vi "USBL_Test.vi"() -> ()   [LabVIEW 2017]
uses:
  <vilib>/Utility/error.llb/DialogType.ctl
  <vilib>/DAQmx/write.llb/DAQmx Write (Analog Wfm 1Chan NSamp).vi
  <vilib>/DAQmx/read.llb/DAQmx Read (Analog 1D Wfm NChan NSamp).vi
  <vilib>/DAQmx/create/channels.llb/DAQmx Create Channel (AO-Voltage-Basic).vi
  <vilib>/DAQmx/configure/events/hardwareSignals.llb/DAQmx Export Signal (Most Signals).vi
  <vilib>/DAQmx/configure/timing.llb/DAQmx Timing (Sample Clock).vi
  <vilib>/DAQmx/miscellaneous.llb/DAQmx Fill In Error Info.vi
  <vilib>/DAQmx/create/channels.llb/DAQmx Create Channel (AI-Voltage-Basic).vi
  <vilib>/DAQmx/configure/trigger.llb/DAQmx Start Trigger (Digital Edge).vi
  <vilib>/Analysis/NI_AALBase.lvlib
panel:
  out "Rx. Signal 9":waveform(dbl)(graph)={"t0"=timestamp(0 s since 1904-01-01), "dt"=1e-05, "Y"=array[100000 elements]}
  out "Rx. Signal 8":waveform(dbl)(graph)={"t0"=timestamp(0 s since 1904-01-01), "dt"=1e-05, "Y"=array[100000 elements]}
  out "Rx. Signal 7":waveform(dbl)(graph)={"t0"=timestamp(0 s since 1904-01-01), "dt"=1e-05, "Y"=array[100000 elements]}
  out "Rx. Signal 6":waveform(dbl)(graph)={"t0"=timestamp(0 s since 1904-01-01), "dt"=1e-05, "Y"=array[100000 elements]}
  out "Rx. Signal 5":waveform(dbl)(graph)={"t0"=timestamp(0 s since 1904-01-01), "dt"=1e-05, "Y"=array[100000 elements]}
  out "Rx. Signal 4":waveform(dbl)(graph)={"t0"=timestamp(0 s since 1904-01-01), "dt"=1e-05, "Y"=array[100000 elements]}
  out "Rx. Signal 3":waveform(dbl)(graph)={"t0"=timestamp(0 s since 1904-01-01), "dt"=1e-05, "Y"=array[100000 elements]}
  out "Rx. Signal 2":waveform(dbl)(graph)={"t0"=timestamp(0 s since 1904-01-01), "dt"=1e-05, "Y"=array[100000 elements]}
  in  "Tx.Channel":tag="PXI1Slot12/ao1"
  in  "Trigger Output":tag="/PXI1Slot12/PFI2"
  in  "Frequency (Hz)":dbl=5000.0
  in  "Amplitude  (V)":dbl=2.5
  in  "Pulse Length (sec)":dbl=0.1
  in  "Device 2":tag="PXI1Slot12"
  out "Rx. Signal":waveform(dbl)[](graph)=[{"t0"=timestamp(3673929480.9649253 s since 1904-01-01), "dt"=9.999999999999972e-06, "Y"=array[10000 elements], "attributes"=variant("NI_ChannelName"=variant(string "PXI1Slot16/ai0"), "NI_UnitDescription"=variant(string "Volts"))}, {"t0"=timestamp(3673929480.9649253 s since 1904-01-01), "dt"=9.999999999999972e-06, "Y"=array[10000 elements], "attributes"=variant("NI_ChannelName"=variant(string "PXI1Slot16/ai1"), "NI_UnitDescription"=variant(string "Volts"))}, {"t0"=timestamp(3673929480.9649253 s since 1904-01-01), "dt"=9.999999999999972e-06, "Y"=array[10000 elements], "attributes"=variant("NI_ChannelName"=variant(string "PXI1Slot16/ai2"), "NI_UnitDescription"=variant(string "Volts"))}, {"t0"=timestamp(3673929480.9649253 s since 1904-01-01), "dt"=9.999999999999972e-06, "Y"=array[10000 elements], "attributes"=variant("NI_ChannelName"=variant(string "PXI1Slot16/ai3"), "NI_UnitDescription"=variant(string "Volts"))}, {"t0"=timestamp(3673929480.9649253 s since 1904-01-01), "dt"=9.999999999999972e-06, "Y"=array[10000 elements], "attributes"=variant("NI_ChannelName"=variant(string "PXI1Slot16/ai4"), "NI_UnitDescription"=variant(string "Volts"))}, {"t0"=timestamp(3673929480.9649253 s since 1904-01-01), "dt"=9.999999999999972e-06, "Y"=array[10000 elements], "attributes"=variant("NI_ChannelName"=variant(string "PXI1Slot16/ai5"), "NI_UnitDescription"=variant(string "Volts"))}, {"t0"=timestamp(3673929480.9649253 s since 1904-01-01), "dt"=9.999999999999972e-06, "Y"=array[10000 elements], "attributes"=variant("NI_ChannelName"=variant(string "PXI1Slot16/ai6"), "NI_UnitDescription"=variant(string "Volts"))}, {"t0"=timestamp(3673929480.9649253 s since 1904-01-01), "dt"=9.999999999999972e-06, "Y"=array[10000 elements], "attributes"=variant("NI_ChannelName"=variant(string "PXI1Slot16/ai7"), "NI_UnitDescription"=variant(string "Volts"))}]
  in  "Number of Sample":i32=10000
  in  "Rx.Time Length (sec)":dbl=1.0
  in  "Trigger Input":tag="/PXI1Slot12/PFI2"
  in  "Sampling Frequency (Hz)":dbl=100000.0
  in  "Rx.Channel":tag="PXI1Slot16/ai0:7"
  in  "Device":tag="PXI1Slot16"
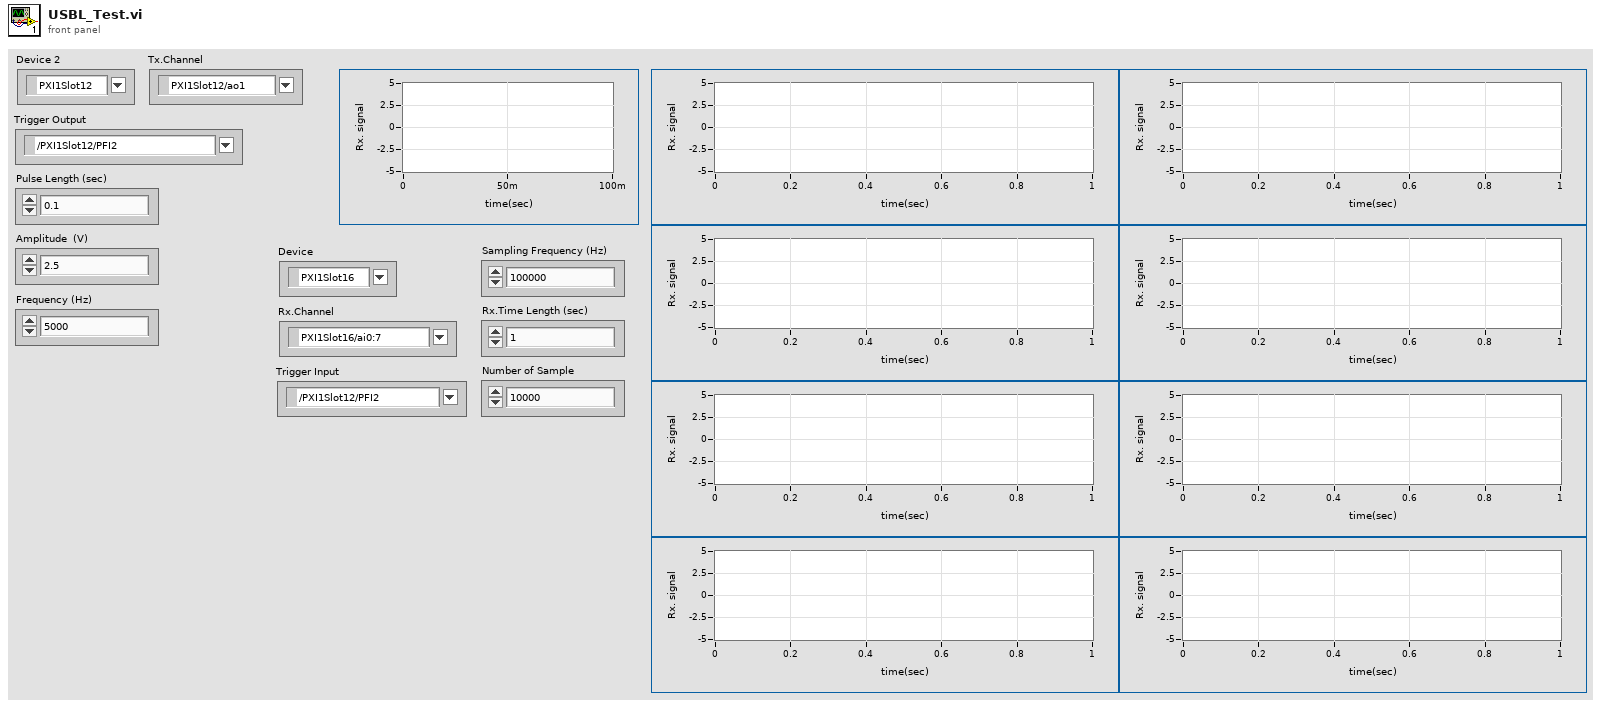
[diagram p1: front panel]
types:
  T1 = typedef "DialogType.ctl" = u16
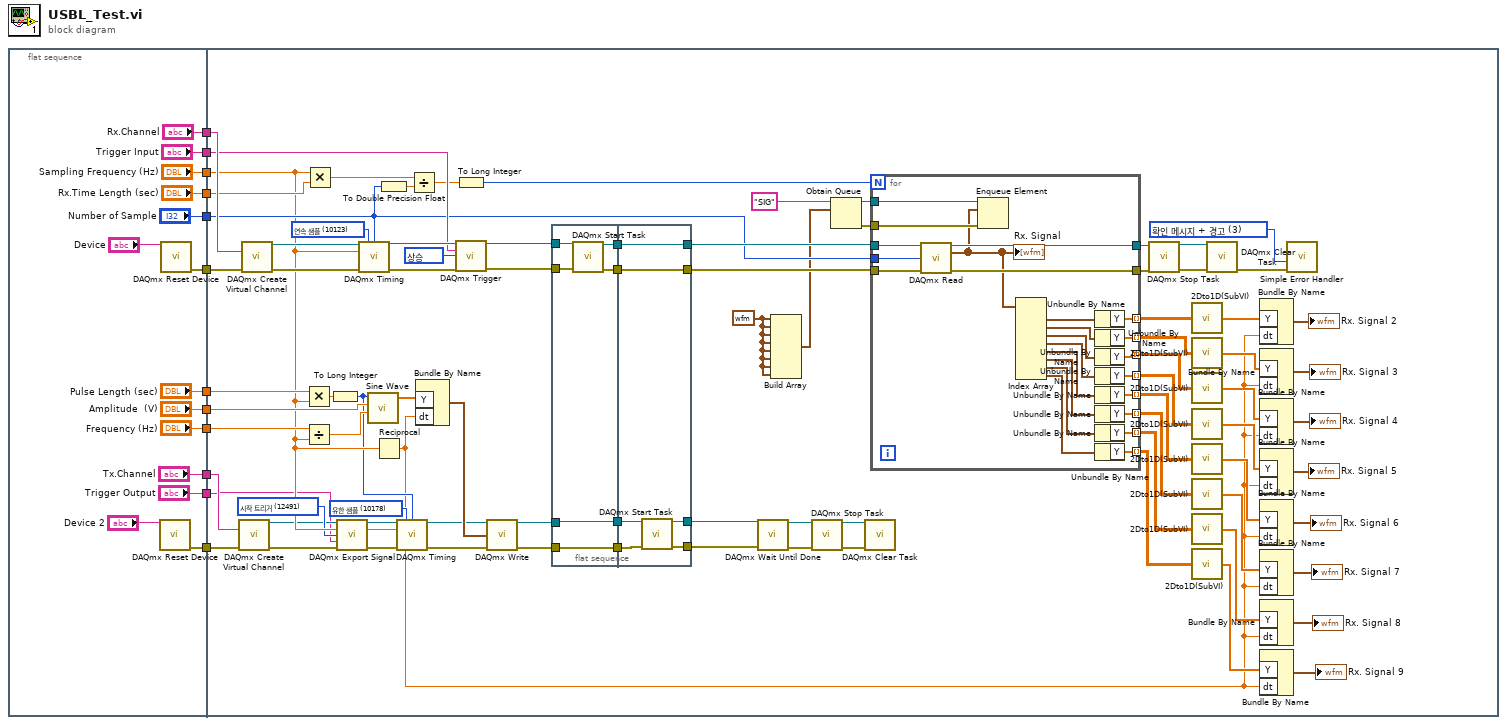
[diagram p0: block diagram]
diagram:
  n1 = flat-sequence {
    tunnel: [w25] -> w12
    tunnel: ["Rx.Channel"] -> w11
    tunnel: ["Trigger Input"] -> w10
    tunnel: ["Sampling Frequency (Hz)"] -> w9
    tunnel: ["Rx.Time Length (sec)"] -> w8
    tunnel: ["Number of Sample"] -> w7
    tunnel: [w18] -> w6
    tunnel: ["Pulse Length (sec)"] -> w5
    tunnel: ["Amplitude  (V)"] -> w4
    tunnel: ["Frequency (Hz)"] -> w3
    tunnel: ["Tx.Channel"] -> w2
    tunnel: ["Trigger Output"] -> w1
    tunnel: w12 -> [w84]
    tunnel: w11 -> [w111]
    tunnel: w10 -> [w108]
    tunnel: w9 -> [w75]
    tunnel: w8 -> [w110]
    tunnel: w7 -> [w97]
    tunnel: w6 -> [w83]
    tunnel: w5 -> [w80]
    tunnel: w4 -> [w79]
    tunnel: w3 -> [w78]
    tunnel: w2 -> [w73]
    tunnel: w1 -> [w63]
    frame #0 {
      n2 = call <vilib>:"DAQmx Reset Device.vi"("device in"="Device 2") -> ("error out"=w18:errorcluster)  [unwired: 14 in]
      n3 = call <vilib>:"DAQmx Reset Device.vi"("device in"="Device") -> ("error out"=w25:errorcluster)  [unwired: 14 in]
    }
    frame #1 {
      w72 = 12491 items=["AI 변환 클럭"=12484, "10MHz 참조 클럭"=12536, "20MHz 타임베이스 클럭"=12486, "샘플 클럭"=12487, "진행 트리거"=12488, "참조 트리거"=12490, "시작 트리거"=12491, "진행 완료 이벤트"=12492, "AI 홀드 완료 이벤트"=12493, "카운터 출력 이벤트"=12494, "변경 감지 이벤트"=12511, "워치독 타이머 만료 이벤트"=12512] ("signal")
      w82 = 10178 items=["유한 샘플"=10178, "연속 샘플"=10123, "하드웨어 타이밍에 의한 단일 포인트"=12522] ("sample mode")
      w87 = T1 3 items=["대화 상자 없음", "확인 메시지", "메시지 지속 또는 정지", "확인 메시지 + 경고", "지속/정지 + 경고"] ("대화 상자 타입 (확인 메시지:1)")
      w92 = waveform(dbl) {"t0"=timestamp(0 s since 1904-01-01), "dt"=1.0, "Y"=[]} ("Waveform")
      w101 = 10123 items=["유한 샘플"=10178, "연속 샘플"=10123, "하드웨어 타이밍에 의한 단일 포인트"=12522] ("sample mode")
      w107 = 10280 items=["상승"=10280, "하강"=10171] ("edge")
      n4 = call-poly <vilib>:"DAQmx Create Virtual Channel.vi"("physical channels"=w73, "error in"=w83) -> ("task out"=w65:refnum<k21>, "error out"=w64:errorcluster)  [unwired: 7 in, 5 out]
      n5 = call-poly <vilib>:"DAQmx Create Virtual Channel.vi"("physical channels"=w111, "error in"=w84) -> ("task out"=w113:refnum<k21>, "error out"=w112:errorcluster)  [unwired: 12 in]
      n6 = Multiply(x=w80, y=w75) -> (x*y=w81:dbl)
      n7 = Divide(x=w78, y=w75) -> (x/y=w77:dbl)
      n8 = Multiply(x=w75, y=w110) -> (x*y=w102:dbl)
      n9 = To Long Integer(number=w81) -> (32bit integer=w60:i32)
      n10 = call-poly <vilib>:"DAQmx Export Signal.vi"("task/channels in"=w65, "signal"=w72, "output terminal"=w63, "error in"=w64) -> ("task out"=w62:refnum<k21>, "error out"=w61:errorcluster)  [unwired: 10 in]
      n11 = call-poly <vilib>:"DAQmx Timing.vi"("task/channels in"=w113, "sample mode"=w101, "samples per channel"=w97, "rate"=w75, "error in"=w112) -> ("task out"=w109:refnum<k21>, "error out"=w106:errorcluster)  [unwired: 9 in]
      n12 = call <vilib>:"Sine Wave.vi"("samples"=w60, "amplitude"=w79, "frequency"=w77) -> ("sine wave"=w76:dbl[])  [unwired: 2 in, 2 out]
      n13 = Reciprocal(x=w75) -> (1/x=w35:dbl)
      n14 = To Double Precision Float(number=w97) -> (double precision float=w103:dbl)
      n15 = call-poly <vilib>:"DAQmx Timing.vi"("task/channels in"=w62, "sample mode"=w82, "samples per channel"=w60, "rate"=w75, "error in"=w61) -> ("task out"=w67:refnum<k21>, "error out"=w66:errorcluster)  [unwired: 2 in, 7 out]
      n16 = Divide(x=w102, y=w103) -> (x/y=w100:dbl)
      n17 = Bundle By Name("Y"=w76, "dt"=w35) -> (w74:waveform(dbl))  [unwired: 1 in]
      n18 = To Long Integer(number=w100) -> (32bit integer=w96:i32)
      n19 = call-poly <vilib>:"DAQmx Trigger.vi"("task/channels in"=w109, "source"=w108, "edge"=w107, "error in"=w106) -> ("task out"=w105:refnum<k21>, "error out"=w104:errorcluster)  [unwired: 10 in]
      n20 = call-poly <vilib>:"DAQmx Write.vi"("task/channels in"=w67, "data"=w74, "error in"=w66) -> ("task out"=w55:refnum<k21>, "error out"=w54:errorcluster)  [unwired: 10 in, 1 out]
      n21 = flat-sequence {
        tunnel: w105 -> [w119]
        tunnel: w104 -> [w118]
        tunnel: [w117] -> w59
        tunnel: [w116] -> w58
        tunnel: w55 -> [w115]
        tunnel: w54 -> [w114]
        tunnel: [w115] -> w53
        tunnel: [w114] -> w52
        tunnel: [w124] -> w98
        tunnel: [w125] -> w99
        tunnel: w59 -> [w125]
        tunnel: w58 -> [w124]
        tunnel: [w123] -> w57
        tunnel: [w122] -> w56
        tunnel: w53 -> [w121]
        tunnel: w52 -> [w120]
        frame #0 {
          n22 = call <vilib>:"DAQmx Start Task.vi"("task/channels in"=w119, "error in"=w118) -> ("task out"=w117:refnum<k21>, "error out"=w116:errorcluster)  [unwired: 12 in]
        }
        frame #1 {
          n23 = call <vilib>:"DAQmx Start Task.vi"("task/channels in"=w121, "error in"=w120) -> ("task out"=w123:refnum<k21>, "error out"=w122:errorcluster)  [unwired: 12 in]
        }
      }
      n24 = call <vilib>:"DAQmx Wait Until Done.vi"("task/channels in"=w57, "error in"=w56) -> ("task out"=w69:refnum<k21>, "error out"=w68:errorcluster)  [unwired: 12 in]
      n25 = Build Array(w92, w92, w92, w92, w92, w92, w92, w92) -> (w91:waveform(dbl)[])
      n26 = call <vilib>:"DAQmx Stop Task.vi"("task/channels in"=w69, "error in"=w68) -> ("task out"=w71:refnum<k21>, "error out"=w70:errorcluster)  [unwired: 12 in]
      n27 = Obtain Queue(name (unnamed)="SIG" ("이름(이름없음)"), element data type=w91) -> (queue out=w93:refnum<queue>, error out=w94:errorcluster)  [unwired: 3 in, 1 out]
      n28 = call <vilib>:"DAQmx Clear Task.vi"("task in"=w71, "error in"=w70) -> ()  [unwired: 13 in, 1 out]
      n29 = for "For 루프" {
        N: w96 -> [_]
        tunnel: w93 -> [w149]
        tunnel: w94 -> [w148]
        tunnel: w99 -> [w147]
        tunnel: w98 -> [w146]
        tunnel: w97 -> [w145]
        tunnel: [w144] -> w86
        tunnel: [w143] -> w85
        tunnel: [w140] -> w51 mode=indexing
        tunnel: [w132] -> w50 mode=indexing
        tunnel: [w131] -> w49 mode=indexing
        tunnel: [w130] -> w48 mode=indexing
        tunnel: [w129] -> w47 mode=indexing
        tunnel: [w128] -> w46 mode=indexing
        tunnel: [w127] -> w45 mode=indexing
        tunnel: [w126] -> w44 mode=indexing
        n30 = call-poly <vilib>:"DAQmx Read.vi"("task/channels in"=w147, "number of samples per channel"=w145, "error in"=w146) -> ("task out"=w144:refnum<k21>, "data"=w142:waveform(dbl)[], "error out"=w143:errorcluster)  [unwired: 10 out]
        "Rx. Signal" <- w142
        n31 = Enqueue Element(queue=w149, element=w142, error in (no error)=w148) -> ()  [unwired: 1 in, 3 out]
        n32 = Index Array(array=w142) -> (element #1=w141:waveform(dbl), element #2=w139:waveform(dbl), element #3=w138:waveform(dbl), element #4=w137:waveform(dbl), element #5=w136:waveform(dbl), element #6=w135:waveform(dbl), element #7=w134:waveform(dbl), element #8=w133:waveform(dbl))  [unwired: 8 in]
        n33 = Unbundle By Name(w141) -> ("Y"=w140:dbl[])
        n34 = Unbundle By Name(w139) -> ("Y"=w132:dbl[])
        n35 = Unbundle By Name(w138) -> ("Y"=w131:dbl[])
        n36 = Unbundle By Name(w137) -> ("Y"=w130:dbl[])
        n37 = Unbundle By Name(w136) -> ("Y"=w129:dbl[])
        n38 = Unbundle By Name(w135) -> ("Y"=w128:dbl[])
        n39 = Unbundle By Name(w134) -> ("Y"=w127:dbl[])
        n40 = Unbundle By Name(w133) -> ("Y"=w126:dbl[])
      }
      n41 = call <vilib>:"DAQmx Stop Task.vi"("task/channels in"=w86, "error in"=w85) -> ("task out"=w90:refnum<k21>, "error out"=w89:errorcluster)  [unwired: 12 in]
      n42 = call "2Dto1D(SubVI).vi"("X1"=w51) -> ("Y1"=w43:dbl[])
      n43 = call "2Dto1D(SubVI).vi"("X1"=w50) -> ("Y1"=w42:dbl[])
      n44 = call "2Dto1D(SubVI).vi"("X1"=w49) -> ("Y1"=w41:dbl[])
      n45 = call "2Dto1D(SubVI).vi"("X1"=w48) -> ("Y1"=w40:dbl[])
      n46 = call "2Dto1D(SubVI).vi"("X1"=w47) -> ("Y1"=w39:dbl[])
      n47 = call "2Dto1D(SubVI).vi"("X1"=w46) -> ("Y1"=w38:dbl[])
      n48 = call "2Dto1D(SubVI).vi"("X1"=w45) -> ("Y1"=w37:dbl[])
      n49 = call "2Dto1D(SubVI).vi"("X1"=w44) -> ("Y1"=w36:dbl[])
      n50 = call <vilib>:"DAQmx Clear Task.vi"("task in"=w90, "error in"=w89) -> ("error out"=w88:errorcluster)  [unwired: 13 in]
      n51 = Bundle By Name("Y"=w43, "dt"=w35) -> (→"Rx. Signal 2":waveform(dbl))  [unwired: 1 in]
      n52 = Bundle By Name("Y"=w42, "dt"=w35) -> (→"Rx. Signal 3":waveform(dbl))  [unwired: 1 in]
      n53 = Bundle By Name("Y"=w41, "dt"=w35) -> (→"Rx. Signal 4":waveform(dbl))  [unwired: 1 in]
      n54 = Bundle By Name("Y"=w40, "dt"=w35) -> (→"Rx. Signal 5":waveform(dbl))  [unwired: 1 in]
      n55 = Bundle By Name("Y"=w39, "dt"=w35) -> (→"Rx. Signal 6":waveform(dbl))  [unwired: 1 in]
      n56 = Bundle By Name("Y"=w38, "dt"=w35) -> (→"Rx. Signal 7":waveform(dbl))  [unwired: 1 in]
      n57 = Bundle By Name("Y"=w37, "dt"=w35) -> (→"Rx. Signal 8":waveform(dbl))  [unwired: 1 in]
      n58 = Bundle By Name("Y"=w36, "dt"=w35) -> (→"Rx. Signal 9":waveform(dbl))  [unwired: 1 in]
      n59 = call <vilib>:"Simple Error Handler.vi"("type of dialog (OK msg:1)"=w87, "error in (no error)"=w88) -> ()  [unwired: 3 in, 5 out]
    }
  }
